vi "Botspeak_HTTP_Init.vi"() -> ()   [LabVIEW 2014]
panel:
  in  "URL":string
  in  "file":path
  out "body":string
  out "headers":string
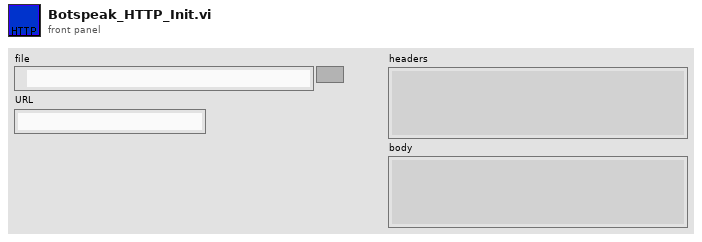
[diagram p1: front panel]
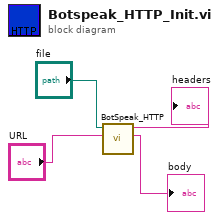
[diagram p0: block diagram]
diagram:
  n1 = call <userlib>:"BotSpeak_HTTP.vi"("URL"="URL", "file"="file") -> ("body"=→"body":string, "headers"=→"headers":string)  [unwired: 8 in]
